vi "1 Parallel Loops.vi"() -> ()   [LabVIEW 2014]
uses:
  <vilib>/Analysis/NI_AALBase.lvlib
panel:
  out "Analysis LED":bool
  in  "Stop Button":bool
  out "Histogram":dynamicdata(graph)
  out "STD":dbl(knob) scale=0.0..100.0
  out "Mean":dbl(knob) scale=0.0..100.0
  out "Thermometer":dbl(slide) scale=0.0..100.0
  out "Waveform Chart":dbl(graph)
  in  "Enable Analysis":bool
  in  "Temp":dbl(knob) scale=0.0..100.0
  # "Parallel Loops (Pahse 1)"
  # "Temperature"
  # "Temperature Log"
  # "Statistics"
  # "Statistics"
  # "Analysis \nStatus"
  # "Exit Program"
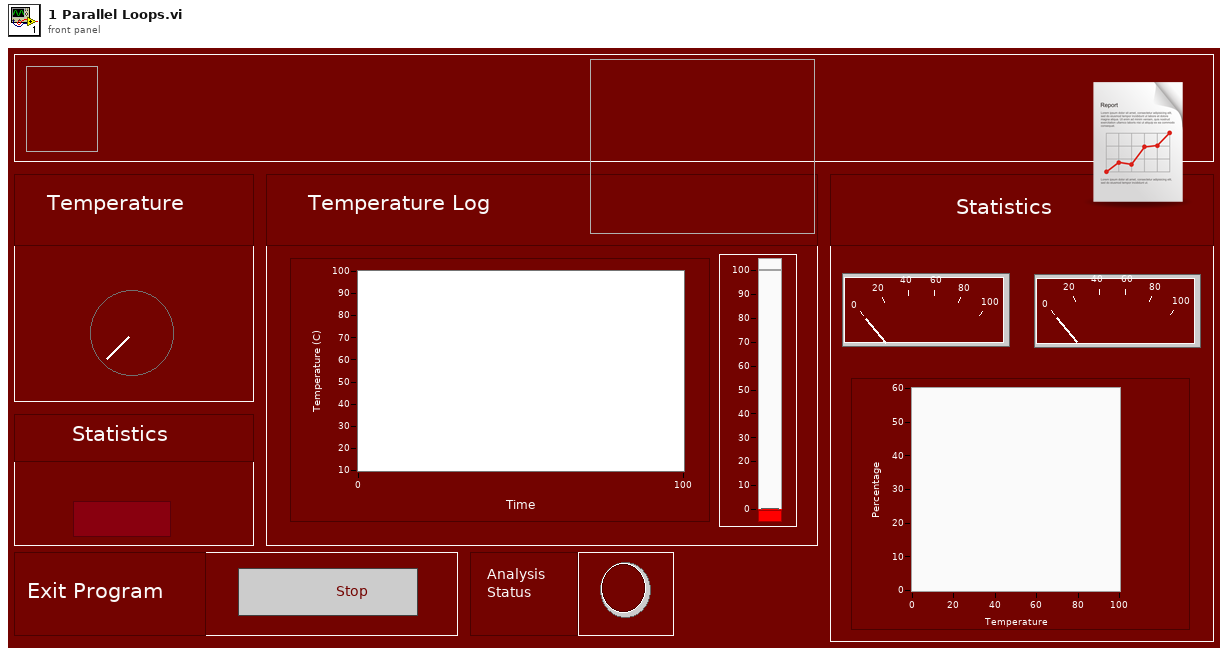
[diagram p1: front panel]
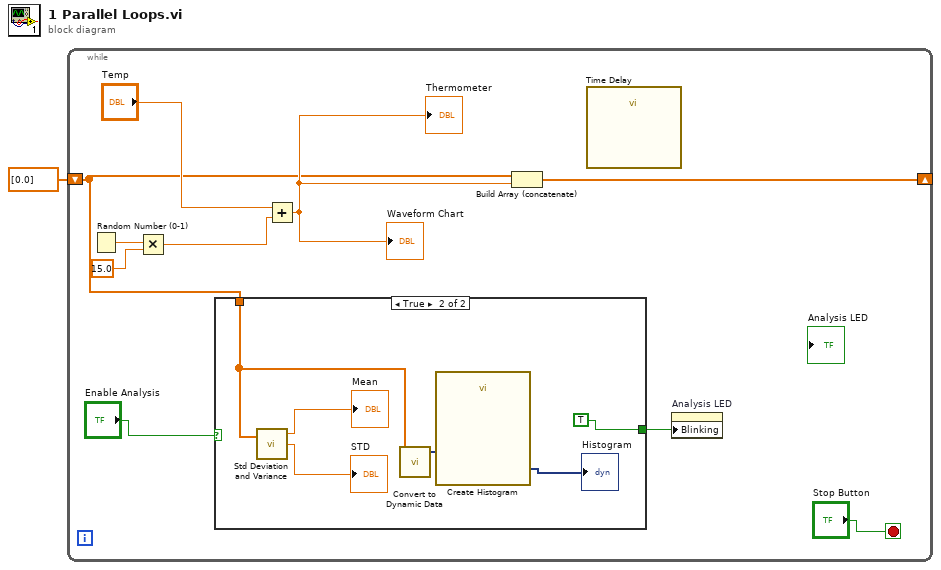
[diagram p0: block diagram]
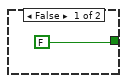
[diagram p2: hidden frame]
diagram:
  n1 = while {
    shift-right: [w5] -> _
    shift-left: dbl[] [0.0] -> [w4]
    stop <- "Stop Button" stop-if-true
    n2 = Random Number (0-1)() -> (number: 0 to 1=w10:dbl)
    n3 = Multiply(x=w10, y=15.0) -> (x*y=w8:dbl)
    n4 = case shown="True" "Enable Analysis" {
      tunnel: w4 -> [_ w16]
      tunnel: [FALSE TRUE] -> w2
      frame False {
      }
      frame True {
        n5 = call <vilib>:"Std Deviation and Variance.vi"("X"=w16) -> ("mean"=→"Mean":dbl, "standard deviation"=→"STD":dbl)  [unwired: 1 in, 1 out]
        n6 = call "Convert to Dynamic Data"("Array"=w16) -> ("Dynamic Data Type"=w15:dynamicdata)  [unwired: 3 in]
        n7 = call "Create Histogram"("Signal"=w15) -> ("Histogram"=→"Histogram":dynamicdata)  [unwired: 9 in, 1 out]
      }
    }
    n8 = Add(x="Temp", y=w8) -> (x+y=w6:dbl)
    "Waveform Chart" <- w6
    "Thermometer" <- w6
    n9 = Build Array (concatenate)(w4, w6) -> (w5:dbl[])
    n10 = call "Time Delay"() -> ()  [unwired: 11 in, 1 out]
    n11 = property on="Analysis LED" class="Bool (strict)"("Blinking"=w2) -> ()  [unwired: 2 in, 2 out]
  }
